vi "find channel.vi"(9 "Channels":string[](array[string]), 10 "Measurement Data":dbl[](array[numeric]), 11 "Measurement Source":T1=enum."T3") -> (3 "element":dbl)   [LabVIEW 2015]
uses:
  Custom Controls/AllSources.ctl
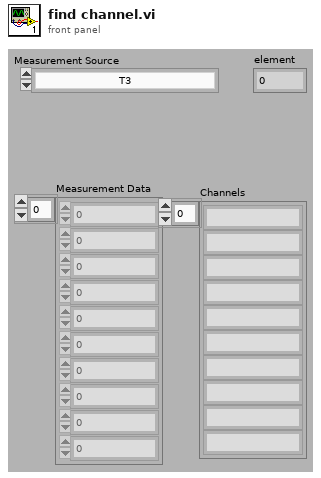
[diagram p1: front panel]
types:
  T1 = typedef "AllSources.ctl" = enum16{"J11.6 VBAT_5A", "TP10 3V3", "TP9 3V", "TP8 2V5", "TP7 1V5", "TP6 1V2", "TP14 AVDD", "TP12 D_VGH", "TP13 D_VGL", "TP11 VFET", "T3", "T4", "T5", "T6", "T7", " IGNITION_DETECT", "T8", "T9", "Low Side Charger Load", "J2004 CH_IF_LOAD", "CAR1", "CAR2", "CAR3", "DMM PIN 24", "RESERVED AND BANNANA", "CAR6", "CAR7", "CAR8", "CAR9", "CAR10", "CAR11", "CAR12", "CAR13", "CAR14", "CAR15", "J3.23 5V_VIC", "DMM PIN37", "VBAT", "DMM PIN 39", "DMM PIN 40"}
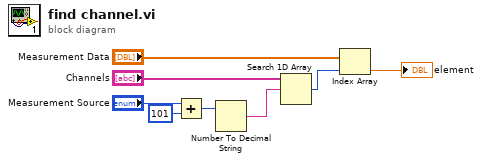
[diagram p0: block diagram]
diagram:
  n1 = Add(x="Measurement Source", y=u16 101) -> (x+y=w6:u16)
  n2 = Number To Decimal String(number=w6) -> (decimal integer string=w4:string)  [unwired: 1 in]
  n3 = Search 1D Array(1D array="Channels", element=w4) -> (index of element=w2:i32)  [unwired: 1 in]
  n4 = Index Array(array="Measurement Data", index=w2) -> (element=→"element":dbl)
